vi "consol_0001_norm_Flash2.vi"() -> ()   [LabVIEW 2022 SP3]
uses:
  <vilib>/Utility/file.llb/Read From Spreadsheet File (DBL).vi
  <vilib>/Utility/file.llb/Write To Spreadsheet File (DBL).vi
panel:
  in  "Path":path=path "C:/Tmp"
  in  "Saving period in seconds":dbl=15.0
  out "Save event":bool caption="Time has Elapsed"
  in  "auto save":bool
  in  "norm":bool=TRUE
  out "XY Graph 2":cluster{"X":dbl[], dbl[]}[](graph)
  out "XF":dbl[](array[numeric])
  out "X":dbl[](array[numeric])
  in  "wavelength\ncoefficients":bool=TRUE
  out "XY Graph":cluster{"X":dbl[], dbl[]}[](graph)
  out "scan":i32
  out "Error":bool
  in  "save":bool
  in  "Fast":bool
  in  "endPix":u16=3652
  in  "startPix":u16
  in  "keep trigger":bool
  in  "blank scans":u8
  in  "scans number":u8=1
  in  "trigger":bool
  out "background":dbl[](array[numeric])
  in  "Substract\nbackground":bool
  in  "N spectra (avrg)":u16=1
  in  "Get Background":bool
  in  "stop":bool
  in  "Exposure (*2.375 ms)":u16=2
  # "Save spectra periodically"
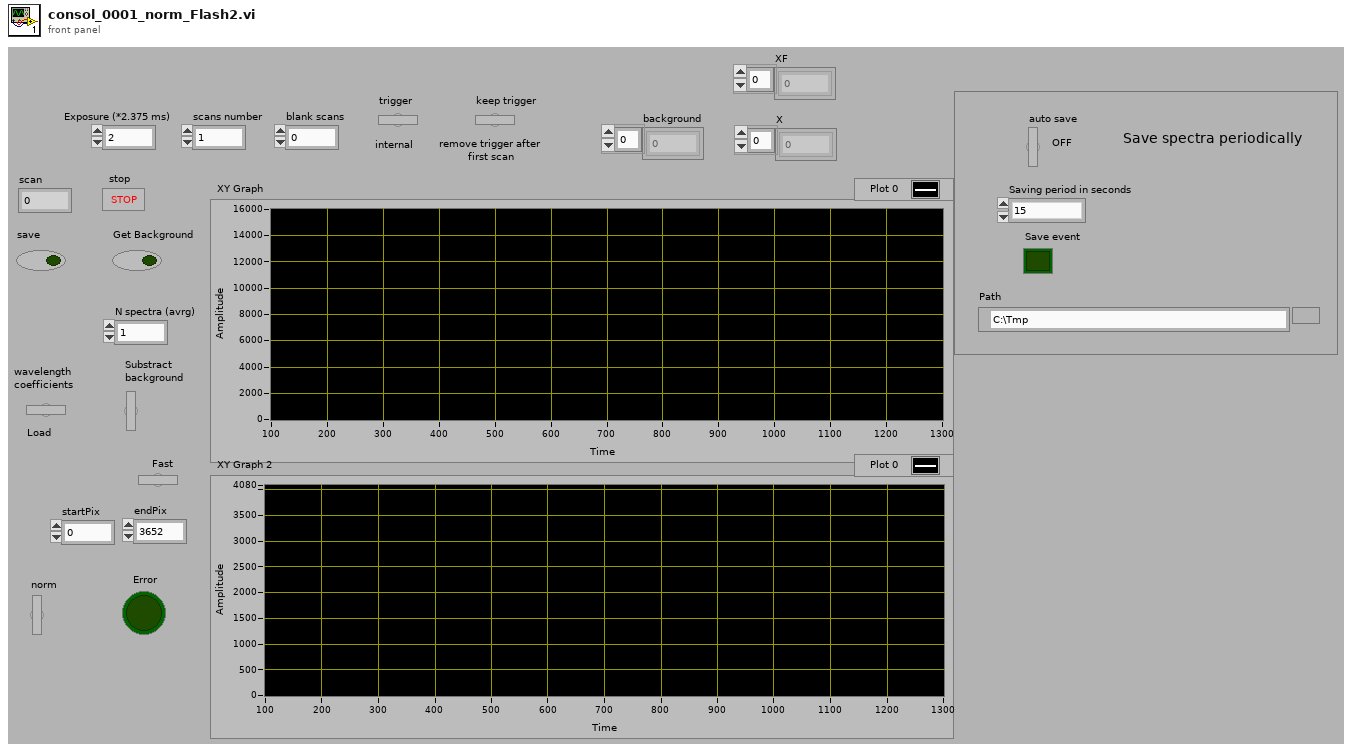
[diagram p1: front panel]
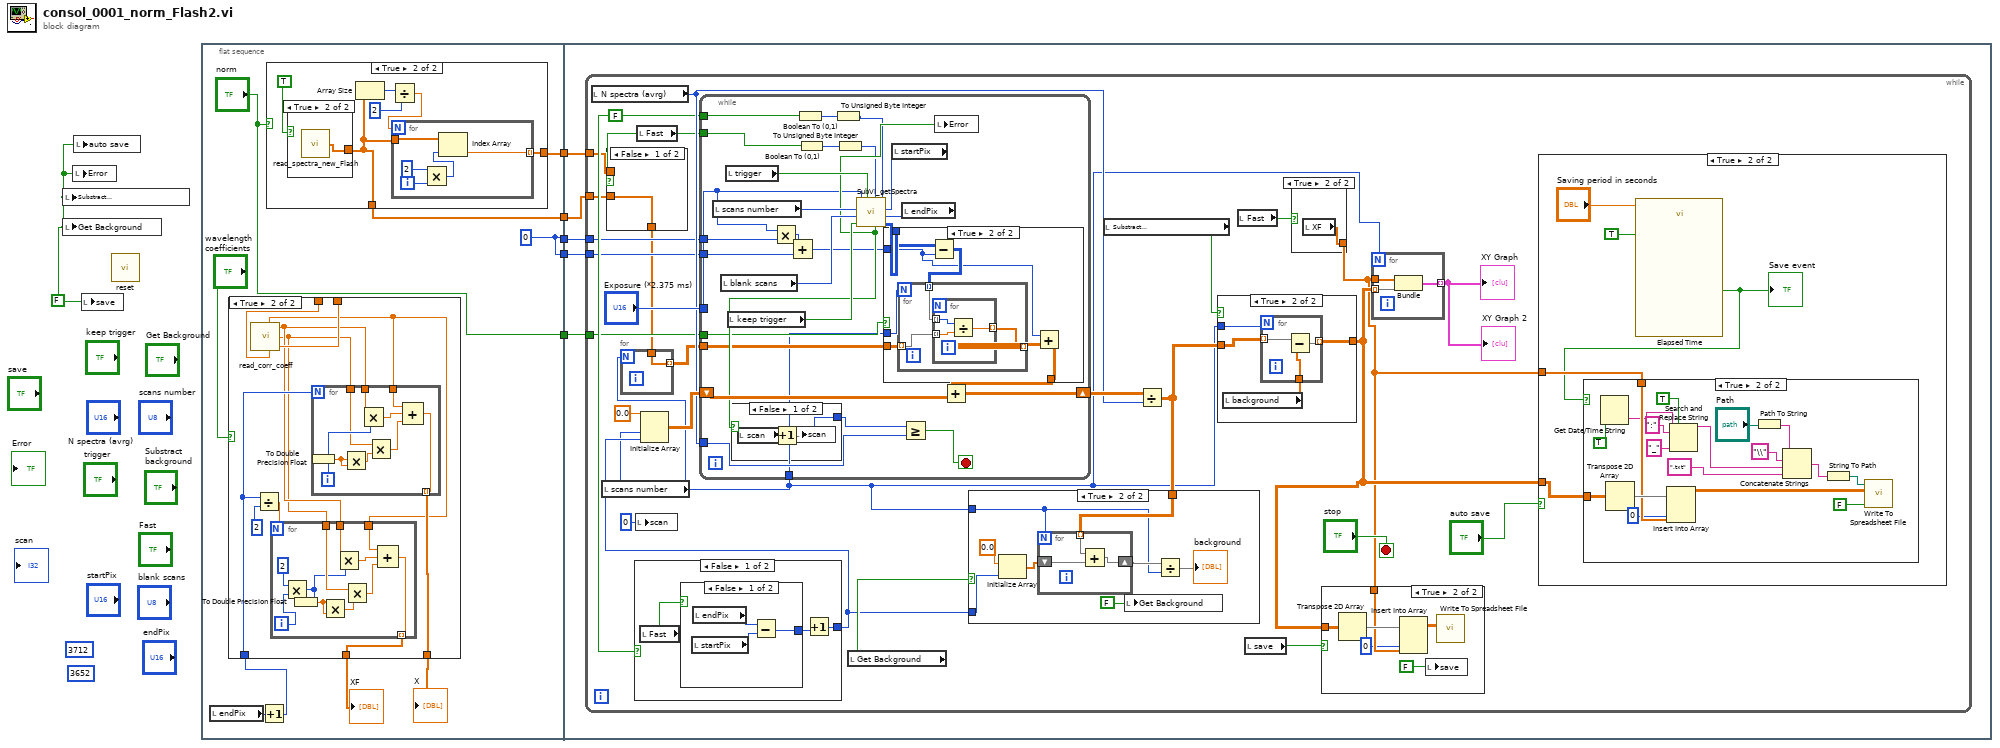
[diagram p0: block diagram]
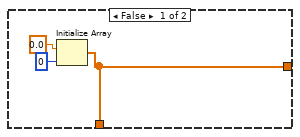
[diagram p2: hidden frame]
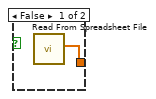
[diagram p3: hidden frame]
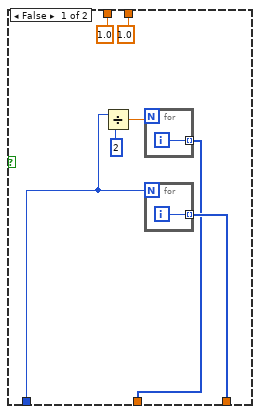
[diagram p4: hidden frame]
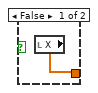
[diagram p8: hidden frame]
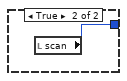
[diagram p10: hidden frame]
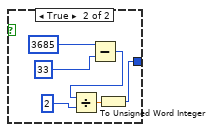
[diagram p12: hidden frame]
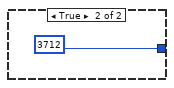
[diagram p13: hidden frame]
diagram:
  (unwired) 3652 ("dimension size")
  (unwired) u16 3712
  w1 = FALSE
  n1 = local write "Substract\nbackground"(w1) -> ()
  n2 = local write "Get Background"(w1) -> ()
  n3 = local write "Error"(w1) -> ()
  n4 = local write "auto save"(w1) -> ()
  n5 = local write "save"(w1) -> ()
  n6 = call "reset.vi"() -> ()  [unwired: 1 in]
  n7 = flat-sequence {
    tunnel: ["norm"] -> w6
    tunnel: [w7] -> w5
    tunnel: [w7] -> w4
    tunnel: [w9] -> w3
    tunnel: [w8] -> w2
    tunnel: w6 -> [w75]
    tunnel: w5 -> [w74]
    tunnel: w4 -> [w73]
    tunnel: w3 -> [w72]
    tunnel: w2 -> [w71]
    frame #0 {
      w7 = 0
      n8 = local read "endPix"() -> (w14:u16)
      n9 = Increment(x=w14) -> (x+1=w13:u16)
      n10 = case shown="True" "wavelength\ncoefficients" {
        tunnel: w13 -> [w36 w48]
        tunnel: [w38 w50] -> w12
        tunnel: [w34 w46] -> w11
        tunnel: [1.0 ("bck: a\n(ax+b)") w44] -> _
        tunnel: [1.0 ("bck: b\n(ax+b)") w45] -> _
        frame False {
          n11 = Divide(x=w36, y=u16 2) -> (x/y=w37:dbl)
          n12 = for {
            N: w37 -> [_]
            tunnel: [w39] -> w34 mode=indexing
            i -> [w39]
          }
          n13 = for {
            N: w36 -> [_]
            tunnel: [w40] -> w38 mode=indexing
            i -> [w40]
          }
        }
        frame True {
          n14 = call "read_corr_coeff.vi"() -> ("bck: a\n(ax+b)"=w44:dbl, "bck: b\n(ax+b)"=w45:dbl, "A\n(Ax^2+Bx+C)"=w41:dbl, "B\n(Ax^2+Bx+C)"=w42:dbl, "C\n(Ax^2+Bx+C)"=w43:dbl)  [unwired: 1 in]
          n15 = Divide(x=w48, y=2) -> (x/y=w49:dbl)
          n16 = for {
            N: w49 -> [_]
            tunnel: w43 -> [w60]
            tunnel: w42 -> [w59]
            tunnel: w41 -> [w58]
            tunnel: [w56] -> w46 mode=indexing
            i -> [w54]
            n17 = Multiply(x=2, y=w54) -> (x*y=w55:i32)
            n18 = To Double Precision Float(number=w55) -> (double precision float=w51:dbl)
            n19 = Multiply(x=w51, y=w51) -> (x*y=w52:dbl)
            n20 = Multiply(x=w59, y=w55) -> (x*y=w61:dbl)
            n21 = Multiply(x=w58, y=w52) -> (x*y=w57:dbl)
            n22 = Compound Arithmetic op=ADD(w60, w61, w57) -> (w56:dbl)
          }
          n23 = for {
            N: w48 -> [_]
            tunnel: w43 -> [w68]
            tunnel: w42 -> [w67]
            tunnel: w41 -> [w66]
            tunnel: [w64] -> w50 mode=indexing
            i -> [w70]
            n24 = To Double Precision Float(number=w70) -> (double precision float=w62:dbl)
            n25 = Multiply(x=w62, y=w62) -> (x*y=w63:dbl)
            n26 = Multiply(x=w67, y=w70) -> (x*y=w69:dbl)
            n27 = Multiply(x=w66, y=w63) -> (x*y=w65:dbl)
            n28 = Compound Arithmetic op=ADD(w68, w69, w65) -> (w64:dbl)
          }
        }
      }
      "X" <- w12
      "XF" <- w11
      n29 = case shown="True" "norm" {
        tunnel: [w16 w20] -> w9
        tunnel: [w16 w19] -> w8
        frame False {
          n30 = Initialize Array(0.0 ("element"), 0 ("dimension size")) -> (w16:dbl[])
        }
        frame True {
          n31 = case shown="True" TRUE {
            tunnel: [w30 w31] -> w19
            frame False {
              n32 = call-poly <vilib>:"Read From Spreadsheet File.vi"() -> ("first row"=w30:dbl[])  [unwired: 7 in, 4 out]
            }
            frame True {
              n33 = call "read_spectra_new_Flash.vi"() -> ("correction"=w31:dbl[])
            }
          }
          n34 = Array Size(array=w19) -> (size(s)=w23:i32)
          n35 = Divide(x=w23, y=2) -> (x/y=w21:dbl)
          n36 = for {
            N: w21 -> [_]
            tunnel: w19 -> [w29]
            tunnel: [w25] -> w20 mode=indexing
            i -> [w28]
            n37 = Multiply(x=2, y=w28) -> (x*y=w27:i32)
            n38 = Index Array(array=w29, index=w27) -> (element=w25:dbl)
          }
        }
      }
    }
    frame #1 {
      n39 = while {
        tunnel: w75 -> [w87]
        tunnel: w74 -> [w84]
        tunnel: w73 -> [w83]
        tunnel: w72 -> [w81]
        tunnel: w71 -> [w80]
        stop <- "stop" stop-if-true
        w89 = FALSE ("Boolean")
        n40 = local read "N spectra (avrg)"() -> (w91:u16)
        n41 = local read "scans number"() -> (w85:u8)
        n42 = case shown="False" w89 {
          tunnel: [w186 u16 3712] -> w94
          frame False {
            n43 = local read "Fast"() -> (w185:bool)
            n44 = case shown="False" w185 {
              tunnel: [w190 w194] -> w187
              frame False {
                n45 = local read "startPix"() -> (w188:u16)
                n46 = local read "endPix"() -> (w189:u16)
                n47 = Subtract(x=w189, y=w188) -> (x-y=w190:u16)
              }
              frame True {
                n48 = Subtract(x=u16 3685, y=u16 33) -> (x-y=w193:u16)
                n49 = Divide(x=w193, y=u16 2) -> (x/y=w195:dbl)
                n50 = To Unsigned Word Integer(number=w195) -> (unsigned 16bit integer=w194:u16)
              }
            }
            n51 = Increment(x=w187) -> (x+1=w186:u16)
          }
          frame True {
          }
        }
        n52 = local write "scan"(0 ("current scan")) -> ()
        n53 = local read "Fast"() -> (w82:bool)
        n54 = case shown="False" w82 {
          tunnel: w81 -> [_ w127]
          tunnel: w80 -> [w126 _]
          tunnel: [w126 w127] -> w79
          frame False {
          }
          frame True {
          }
        }
        n55 = for {
          N: w85 -> [_]
          tunnel: w79 -> [w128]
          tunnel: [w128] -> w86 mode=indexing
        }
        n56 = Initialize Array(0.0 ("element"), w85, w94) -> (w99:dbl[][])
        n57 = while {
          tunnel: "Exposure (*2.375 ms)" -> [w138]
          shift-right: [w160] -> w95
          shift-left: w99 -> [w161]
          tunnel: w91 -> [w150]
          tunnel: w89 -> [w145]
          tunnel: w87 -> [w144]
          tunnel: w86 -> [w143]
          tunnel: w85 -> [w141]
          tunnel: w84 -> [w136]
          tunnel: w83 -> [w135]
          tunnel: w82 -> [w134]
          stop <- w152 stop-if-true
          n58 = local read "scans number"() -> (w158:u8)
          n59 = local read "blank scans"() -> (w157:u8)
          n60 = local read "trigger"() -> (w159:bool)
          n61 = local read "keep trigger"() -> (w156:bool)
          n62 = Multiply(x=w138, y=w136) -> (x*y=w137:i32)
          n63 = Add(x=w137, y=w135) -> (x+y=w139:i32)
          n64 = Boolean To (0,1)(Boolean=w145) -> (0, 1=w147:i16)
          n65 = Boolean To (0,1)(Boolean=w134) -> (0, 1=w149:i16)
          n66 = To Unsigned Byte Integer(number=w147) -> (unsigned 8bit integer=w146:u8)
          n67 = To Unsigned Byte Integer(number=w149) -> (unsigned 8bit integer=w148:u8)
          n68 = local read "startPix"() -> (w154:u16)
          n69 = local read "endPix"() -> (w155:u16)
          n70 = call "SubVI_getSpectra.vi"("endPix"=w155, "startPix"=w154, "test1"=w146, "Fast"=w148, "trigger"=w159, "keep trigger"=w156, "blank scans number"=w157, "scans number"=w158, "Exposure"=w138) -> ("all spectra"=w142:i16[][], "Error"=w153:bool)  [unwired: 1 in]
          n71 = case shown="False" w153 {
            tunnel: [w176 w178] -> w151
            frame False {
              n72 = local read "scan"() -> (w177:i32)
              n73 = Increment(x=w177) -> (x+1=w176:i32)
              n74 = local write "scan"(w176) -> ()
            }
            frame True {
              n75 = local read "scan"() -> (w178:i32)
            }
          }
          n76 = case shown="True" w144 {
            tunnel: w143 -> [_ w166]
            tunnel: w142 -> [w162 w169]
            tunnel: w141 -> [_ w167]
            tunnel: [w162 w164] -> w140
            tunnel: w139 -> [_ w163]
            frame False {
            }
            frame True {
              n77 = Subtract(x=w169, y=w163) -> (x-y=w168:i32[][])
              n78 = for {
                N: w167 -> [_]
                tunnel: w168 -> [w172] mode=indexing
                tunnel: w166 -> [w171] mode=indexing
                tunnel: [w170] -> w165 mode=indexing
                n79 = for {
                  tunnel: w172 -> [w175] mode=indexing
                  tunnel: w171 -> [w174] mode=indexing
                  tunnel: [w173] -> w170 mode=indexing
                  n80 = Divide(x=w175, y=w174) -> (x/y=w173:dbl)
                }
              }
              n81 = Add(x=w163, y=w165) -> (x+y=w164:dbl[][])
            }
          }
          n82 = Greater Or Equal?(x=w151, y=w150) -> (x >= y?=w152:bool)
          n83 = local write "Error"(w153) -> ()
          n84 = Add(x=w140, y=w161) -> (x+y=w160:dbl[][])
        }
        n85 = local read "Get Background"() -> (w98:bool)
        n86 = local read "Substract\nbackground"() -> (w97:bool)
        n87 = Divide(x=w95, y=w91) -> (x/y=w96:dbl[][])
        n88 = case shown="True" w98 {
          tunnel: w96 -> [_ w212]
          tunnel: w85 -> [_ w208]
          tunnel: w94 -> [_ w206]
          frame False {
          }
          frame True {
            n89 = Initialize Array(0.0 ("element"), w206) -> (w210:dbl[])
            n90 = for {
              N: w208 -> [_]
              tunnel: w212 -> [w215] mode=indexing
              shift-right: [w214] -> w209
              shift-left: w210 -> [w216]
              n91 = Add(x=w215, y=w216) -> (x+y=w214:dbl[])
            }
            n92 = local write "Get Background"(FALSE ("Get Background")) -> ()
            n93 = Divide(x=w209, y=w208) -> (x/y=→"background":dbl[])
          }
        }
        n94 = case shown="True" w97 {
          tunnel: w96 -> [w198 w202]
          tunnel: [w198 w200] -> w77
          tunnel: w85 -> [_ w199]
          frame False {
          }
          frame True {
            n95 = local read "background"() -> (w201:dbl[])
            n96 = for {
              N: w199 -> [_]
              tunnel: w202 -> [w205] mode=indexing
              tunnel: w201 -> [w204]
              tunnel: [w203] -> w200 mode=indexing
              n97 = Subtract(x=w205, y=w204) -> (x-y=w203:dbl[])
            }
          }
        }
        n98 = local read "Fast"() -> (w90:bool)
        n99 = local read "save"() -> (w93:bool)
        n100 = case shown="True" w90 {
          tunnel: [w129 w130] -> w76
          frame False {
            n101 = local read "X"() -> (w129:dbl[])
          }
          frame True {
            n102 = local read "XF"() -> (w130:dbl[])
          }
        }
        n103 = case shown="True" w93 {
          tunnel: w77 -> [_ w183]
          tunnel: w76 -> [_ w180]
          frame False {
          }
          frame True {
            n104 = Transpose 2D Array(2D array=w183) -> (transposed array=w181:dbl[][])
            n105 = Insert Into Array(array=w181, index (col)=0 ("disabled index (col)"), new element=w180) -> (w182:dbl[][])  [unwired: 1 in]
            n106 = local write "save"(FALSE) -> ()
            n107 = call-poly <vilib>:"Write To Spreadsheet File.vi"("2D data"=w182) -> ()  [unwired: 7 in, 1 out]
          }
        }
        n108 = for {
          N: w85 -> [_]
          tunnel: w76 -> [w133]
          tunnel: [w132] -> w88 mode=indexing
          tunnel: w77 -> [w131] mode=indexing
          n109 = Bundle("XF"=w133, w131) -> (w132:cluster{"XF":dbl[], dbl[]})  [unwired: 1 in]
        }
        "XY Graph" <- w88
        "XY Graph 2" <- w88
        n110 = case shown="True" "auto save" {
          tunnel: w77 -> [_ w105]
          tunnel: w76 -> [_ w104]
          frame False {
          }
          frame True {
            n111 = call "Elapsed Time"("Time Target (s)"="Saving period in seconds", "Auto Reset"=TRUE) -> ("Time has Elapsed"=w103:bool)  [unwired: 10 in, 7 out]
            "Save event" <- w103
            n112 = case shown="True" w103 {
              tunnel: w105 -> [_ w125]
              tunnel: w104 -> [_ w122]
              frame False {
              }
              frame True {
                n113 = Get Date/Time String(want seconds? (F)=TRUE) -> (time string=w113:string)  [unwired: 2 in, 1 out]
                n114 = Transpose 2D Array(2D array=w125) -> (transposed array=w123:dbl[][])
                n115 = Insert Into Array(array=w123, index (col)=0 ("disabled index (col)"), new element=w122) -> (w124:dbl[][])  [unwired: 1 in]
                n116 = Search and Replace String(replace all?=TRUE ("replace all? (F)"), input string=w113, search string=":", replace string="_" ("replace string (\"\")")) -> (result string=w112:string)  [unwired: 4 in, 3 out]
                n117 = Path To String(path="Path") -> (string=w115:string)
                n118 = Concatenate Strings(w115, "\\" ("string"), w112, ".txt" ("string")) -> (w119:string)
                n119 = String To Path(string=w119) -> (path=w118:path)
                n120 = call-poly <vilib>:"Write To Spreadsheet File.vi"("append to file? (new file:F)"=FALSE, "2D data"=w124, "file path (dialog if empty)"=w118) -> ()  [unwired: 5 in, 1 out]
              }
            }
          }
        }
      }
    }
  }
